vi "Get Name (Instance).vi"(8 "error in (no error)":errorcluster, 11 "System Actor in":refnum<class "System Actor.lvclass">) -> (0 "error out":errorcluster, 2 "System Name - Instance":string, 3 "System Actor out":refnum<class "System Actor.lvclass">)   [LabVIEW 2014, in "Robot Actor Framework.lvlib" / "System Actor.lvlib" / "System Actor.lvclass"]
uses:
  System Actor.lvclass
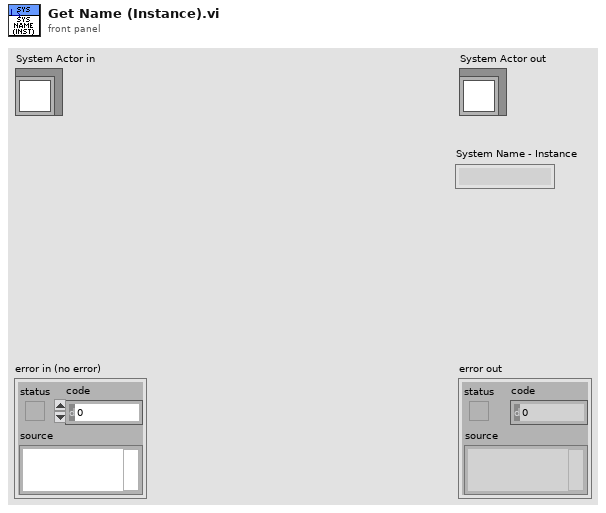
[diagram p1: front panel]
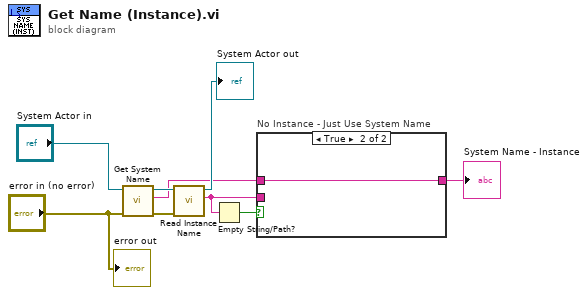
[diagram p0: block diagram]
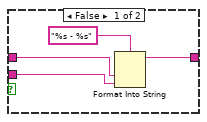
[diagram p2: hidden frame]
diagram:
  n1 = call-dynamic "Get System Name.vi"("error in (no error)"="error in (no error)", "System Actor in"="System Actor in") -> ("error out"=w6:errorcluster, "System Name"=w2:string, "System Actor out"=w5:refnum<class "System Actor.lvclass">)  [unwired: 7 in]
  n2 = call-dynamic "Read Instance Name.vi"("error in (no error)"=w6, "System Actor in"=w5) -> ("Instance Name"=w1:string, "System Actor out"=→"System Actor out":refnum<class "System Actor.lvclass">)  [unwired: 7 in, 1 out]
  n3 = Empty String/Path?(string/path=w1) -> (empty?=w4:bool)
  n4 = case "No Instance - Just Use System Name" shown="True" w4 {
    tunnel: [w13 w14] -> w3
    tunnel: w2 -> [w11 w14]
    tunnel: w1 -> [w10 _]
    frame False {
      n5 = Format Into String(format string="%s - %s", w11, w10) -> (resulting string=w13:string)  [unwired: 2 in, 1 out]
    }
    frame True {
    }
  }
  "System Name - Instance" <- w3
  "error out" <- "error in (no error)"
